vi "Read last Log Value in GroupChannel.vi"() -> ()   [LabVIEW 2011]
panel:
  out "Last Right Value in File":dbl
  out "data R":dbl[](array[numeric])
  out "Last Left Value in File":dbl
  out "data L":dbl[](array[numeric])
  out "Channel Length":i32
  out "found":bool
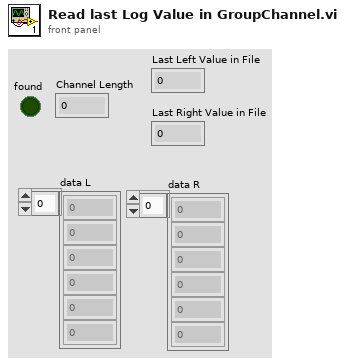
[diagram p1: front panel]
types:
  T1 = enum16{"open", "open or create", "create or replace", "create", "open (read-only)"}
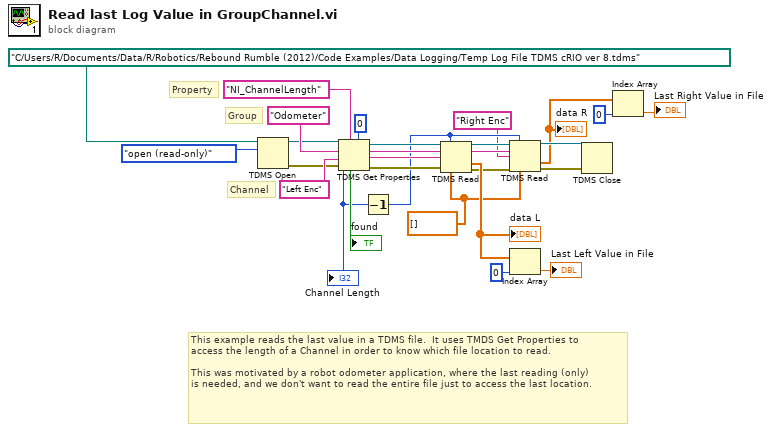
[diagram p0: block diagram]
diagram:
  w6 = dbl[] []
  # "Channel"
  # "Group"
  # "Property"
  # "This example reads the last value in a TDMS file.  It uses TMDS Get Properties to \naccess the length of a Channel in order to know which file location to read. \n\nThis was motivated by a robot odometer application, where the last reading (only) \nis needed, and we don't want to read the entire file just to access the last location."
  n1 = TDMS Open(10:T1."open (read-only)" ("operation (0:open)"), 11:path "C:/Users/R/Documents/Data/R/Robotics/Rebound Rumble (2012)/Code Examples/Data Logging/Temp Log File TDMS cRIO ver 8.tdms" ("file path")) -> (0:w16:errorcluster, 3:w14:refnum<k34>)  [unwired: 4 in]
  n2 = TDMS Get Properties(5:0, 7:"NI_ChannelLength" ("property name"), 8:w16, 9:"Left Enc" ("channel name"), 10:"Odometer" ("group name"), 11:w14) -> (0:w15:errorcluster, 1:w21:string, 2:w22:string, 3:w20:refnum<k34>, 4:w13:i32, 6:→"found":bool)
  "Channel Length" <- w13
  n3 = Decrement(x=w13) -> (x-1=w7:i32)
  n4 = TDMS Read(0:w20, 1:w7, 5:w22, 7:w21, 11:w15, 12:w6) -> (4:w11:refnum<k34>, 6:w5:string, 10:w12:dbl[], 15:w9:errorcluster)  [unwired: 2 in, 2 out]
  "data L" <- w12
  n5 = TDMS Read(0:w11, 1:w7, 5:w5, 7:"Right Enc" ("channel name(s) in"), 11:w9, 12:w6) -> (4:w10:refnum<k34>, 10:w1:dbl[], 15:w8:errorcluster)  [unwired: 2 in, 3 out]
  "data R" <- w1
  n6 = Index Array(array=w12, index=0) -> (element=→"Last Left Value in File":dbl)
  n7 = TDMS Close(8:w8, 11:w10) -> ()  [unwired: 2 out]
  n8 = Index Array(array=w1, index=0) -> (element=→"Last Right Value in File":dbl)
